vi "GOMDBTS2048 calib Measure Spectral.vi"(8 "error in (no error)":errorcluster, 11 "handle":i32) -> (0 "error out":errorcluster, 1 "countsSignal":dbl[](array[numeric]), 2 "countsDark":dbl[](array[numeric]), 3 "saturation":dbl, 4 "function return":i32, 5 "calFactors":dbl[](array[numeric]))   [LabVIEW 2015, in "GOMDBTS2048.lvlib"]
doc: "GOBTS2048DLL int __stdcall GOMDBTS2048_calibMeasureSpectral(int handle, double* saturation, double* countsDark, double* countsSignal, double* calFactors);"
uses:
  GOMDBTS2048.lvlib
  runtime/GOMDBTS2048.dll
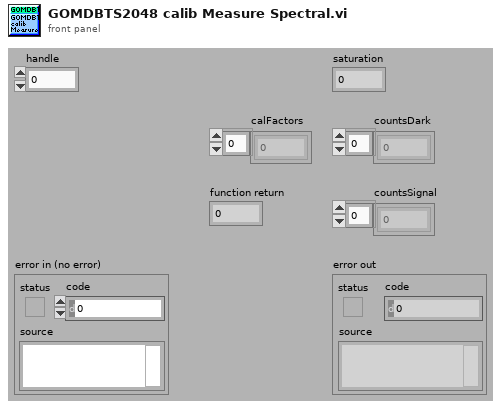
[diagram p1: front panel]
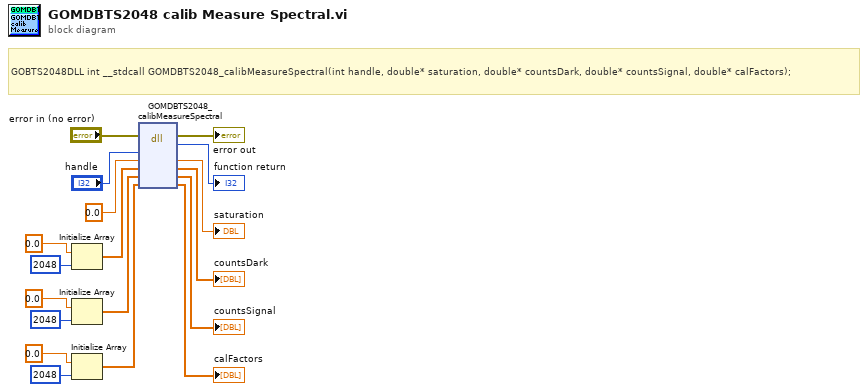
[diagram p0: block diagram]
diagram:
  # "GOBTS2048DLL int __stdcall GOMDBTS2048_calibMeasureSpectral(int handle, double* saturation, double* countsDark, double* countsSignal, double* calFactors);"
  n1 = Initialize Array(0.0 ("element"), 2048 ("dimension size")) -> (w14:dbl[])
  n2 = Initialize Array(0.0 ("element"), 2048 ("dimension size")) -> (w10:dbl[])
  n3 = Initialize Array(0.0 ("element"), 2048 ("dimension size")) -> (w6:dbl[])
  n4 = dll-call lib="C:/Users/rkoch/Documents/GO_Library/runtime/GOMDBTS2048.*" fn="GOMDBTS2048_calibMeasureSpectral"(error in="error in (no error)", "handle"="handle", "saturation"=0.0, "countsDark"=w14, "countsSignal"=w10, "calFactors"=w6) -> (error out=→"error out":errorcluster, "return type"=→"function return":i32, "saturation"=→"saturation":dbl, "countsDark"=→"countsDark":dbl[], "countsSignal"=→"countsSignal":dbl[], "calFactors"=→"calFactors":dbl[])  [unwired: 3 in, 1 out]
